vi "AdcConversion.vi"(8 "error in (no error)":errorcluster, 11 "Conversion in":refnum<class "Conversion.lvclass">) -> (0 "error out":errorcluster, 2 "ADC U8 Array":u8[](array[numeric]), 3 "Conversion out":refnum<class "Conversion.lvclass">)   [LabVIEW 2023, in "Conversion.lvclass"]
doc: "This Conversion class method, converts the analog data to digital data based on the overriding class either by single channel ADC or Multi Channel ADC."
uses:
  Conversion.lvclass
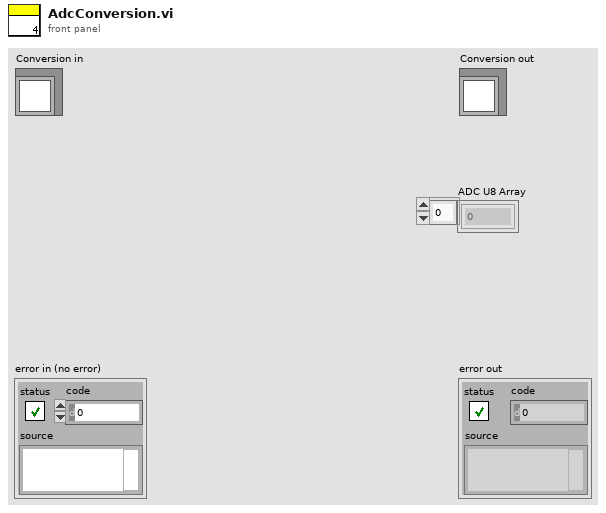
[diagram p1: front panel]
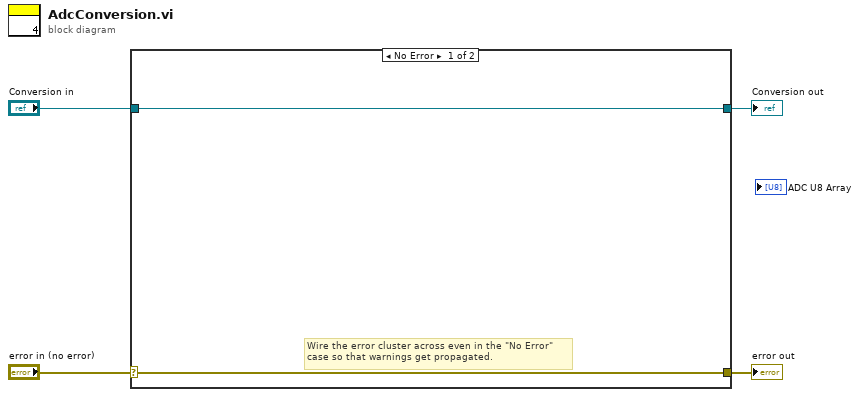
[diagram p0: block diagram]
diagram:
  n1 = case shown="No Error" "error in (no error)" {
    selector: "error in (no error)" -> [w5 w8]
    tunnel: [w5 w8] -> w3
    tunnel: [w6 w7] -> w1
    tunnel: "Conversion in" -> [w6 w7]
    frame No Error {
      # "Wire the error cluster across even in the \"No Error\"\ncase so that warnings get propagated."
    }
    frame Error {
    }
  }
  "error out" <- w3
  "Conversion out" <- w1
